vi "Execute_remote_call.vi"(0 "Traverse line":T4 {"Carrier_2 Q (l/min)" format="%#.2f"; "Row Duration (mins)" format="%#.1f"; "Row No" min=0; "Trace Gas Concentration (%)" min=0.0 format="%#_4f"; "Carrier_1 Q (l/min)" format="%#.4f"; "Start X" format="%#.2f"; "Start Y" format="%#.2f"; "Start Z" format="%#.2f"; "End X" format="%#.2f"; "End Y" format="%#.2f"; "End Z" format="%#.2f"; "Tunnel Speed" format="%#.2f"; "Averaging time (mins)" min=0.0 format="%#.2f"}, 2 "Simulate/Run":T3, 3 "VI to run":path) -> (6 "Traverse Out":T4 {"Carrier_2 Q (l/min)" format="%#.2f"; "Row Duration (mins)" format="%#.1f"; "Row No" min=0; "Trace Gas Concentration (%)" min=0.0 format="%#_4f"; "Carrier_1 Q (l/min)" format="%#.4f"; "Start X" format="%#.2f"; "Start Y" format="%#.2f"; "Start Z" format="%#.2f"; "End X" format="%#.2f"; "End Y" format="%#.2f"; "End Z" format="%#.2f"; "Tunnel Speed" format="%#.2f"; "Averaging time (mins)" min=0.0 format="%#.2f"}, 7 "Status":T2, 8 "Error Messages":string)   [LabVIEW 2020]
uses:
  Traverse_cluster.ctl
  Spacing.ctl
  Controls/Multi_run_mode.ctl
  Controls/User_Specific_mode.ctl
  Multi_Run_Status.ctl
  Controls/Multirun_Execute_Row_Connector_Pane.ctl
panel:
  in  "User Specific":T1
  # "X           Y          Z"
  # "Start"
  # "End"
  # "X           Y          Z"
  # "Start"
  # "End"
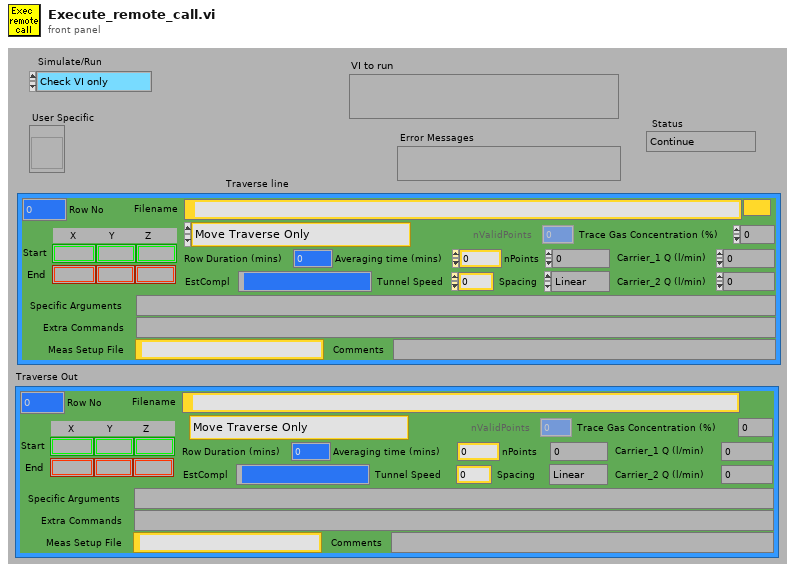
[diagram p1: front panel]
types:
  T1 = typedef "Multirun_Execute_Row_Connector_Pane.ctl" = refnum<vi>
  T2 = typedef "Multi_Run_Status.ctl" = enum16{"Continue", "Continue with Error", "Jump to Next Point", "Jump to Next Row", "Jump To Fall Back", "Terminate Run"}
  T3 = typedef "User_Specific_mode.ctl" = enum16{"Check VI only", "Run VI"}
  T4 = typedef "Traverse_cluster.ctl" = cluster{"Start X":sgl, "Start Y":sgl, "Start Z":sgl, "End X":sgl, "End Y":sgl, "End Z":sgl, "nPoints":i32, "Spacing":T5, "Filename":path, "Tunnel Speed":dbl, "Averaging time (mins)":dbl, "Extra Commands":string, "Carrier_1 Q (l/min)":dbl, "Carrier_2 Q (l/min)":dbl, "Trace Gas Concentration (%)":dbl, "Specific Arguments":string, "Comments":string, "Row No":i32, "Row Type Selector":T6, "EstCompl":string, "Row Duration (mins)":dbl, "nValidPoints":i32, "Meas Setup File":string}
  T5 = typedef "Spacing.ctl" = enum16{"Linear", "Log", "Gauss", "Specified", "N/A"}
  T6 = typedef "Multi_run_mode.ctl" = enum16{"Move Traverse Only", "Set Tunnel Speed Only", "Set Source Only", "Set Measurement Conditions", "Single Measurement", "Vertical Profile", "Lateral Profile", "Longitudinal Profile", "Multi-Axis Profile", "Explore Volume", "Auto Calibrate", "Meas Fast FID Bkgnd", "Check Beam Power", "Scanning Valve Measurement", "Run VI Named:", "Set ADAM Ch", "Wait (minutes)", "Send Message", "Synchronize With:", "Fall Back to this Row", "Turn Off Row Repeating", "Traverse 3D Volume", "Blank Row", "Jump to Fall Back Row"}
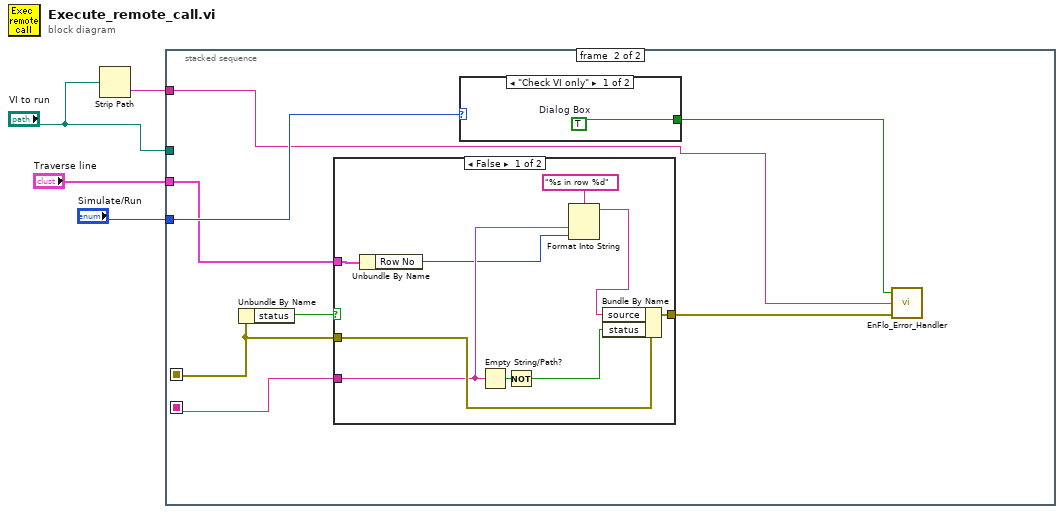
[diagram p0: block diagram]
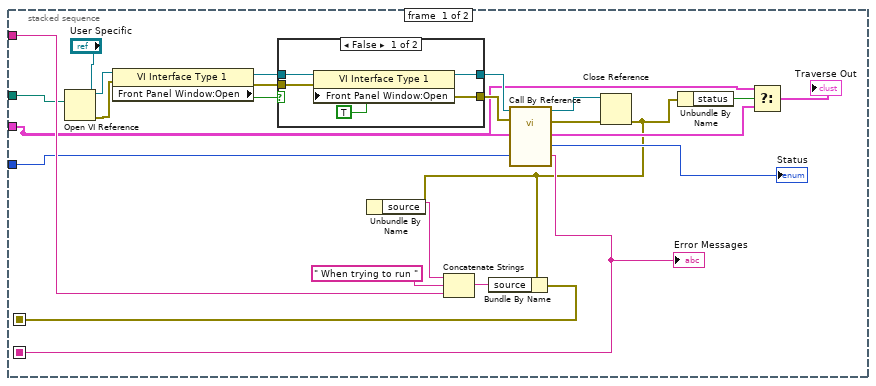
[diagram p2: hidden frame]
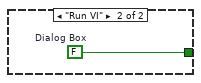
[diagram p4: hidden frame]
diagram:
  n1 = Strip Path(path="VI to run") -> (name=w2:string)  [unwired: 1 out]
  n2 = stacked-sequence {
    seq-local: [w20 _] -> [_ w38]
    seq-local: [w23 _] -> [_ w39]
    tunnel: w2 -> [w24 w36]
    tunnel: "Simulate/Run" -> [w22 w42]
    tunnel: "VI to run" -> [w21 _]
    tunnel: "Traverse line" -> [w6 w37]
    frame #0 {
      n3 = Open VI Reference(type specifier VI Refnum (for type only)="User Specific", vi path=w21) -> (vi reference=w8:T1, error out=w10:errorcluster)  [unwired: 2 in, 2 out]
      n4 = property class="VI Interface Type 1"(reference=w8, error in=w10) -> (reference out=w12:T1, error out=w13:errorcluster, "Front Panel Window:Open"=w11:bool)
      n5 = case shown="False" w11 {
        tunnel: w12 -> [w33 w35]
        tunnel: w13 -> [w32 w34]
        tunnel: [w31 w35] -> w7
        tunnel: [w29 w34] -> w9
        frame False {
          n6 = property class="VI Interface Type 1"(reference=w33, error in=w32, "Front Panel Window:Open"=TRUE) -> (reference out=w31:T1, error out=w29:errorcluster)
        }
        frame True {
        }
      }
      n7 = call-by-ref "?"(reference=w7, error in=w9, "Mode"=w22, "Traverse line In"=w6) -> (reference out=w25:T1, error out=w15:errorcluster, "Error Message"=w20:string, "Status"=→"Status":T2, "Traverse line Out"=w17:T4)  [unwired: 1 in]
      "Error Messages" <- w20
      n8 = Close Reference(reference=w25, error in (no error)=w15) -> (error out=w14:errorcluster)
      n9 = Unbundle By Name(w14) -> ("source"=w28:string)
      n10 = Concatenate Strings(w28, " When trying to run " ("Substring"), w24) -> (w26:string)
      n11 = Bundle By Name(cluster=w14, "source"=w26) -> (w23:errorcluster)
      n12 = Unbundle By Name(w14) -> ("status"=w18:bool)
      n13 = Select(t=w6, s=w18, f=w17) -> (s? t:f=→"Traverse Out":T4)
    }
    frame #1 {
      n14 = Unbundle By Name(w39) -> ("status"=w43:bool)
      n15 = case shown="False" w43 {
        tunnel: [w53 w55] -> w40
        tunnel: w39 -> [w54 w55]
        tunnel: w38 -> [w51 _]
        tunnel: w37 -> [w48 _]
        frame False {
          n16 = Unbundle By Name(w48) -> ("Row No"=w46:i32)
          n17 = Empty String/Path?(string/path=w51) -> (empty?=w52:bool)
          n18 = Not(x=w52) -> (.not. x?=w47:bool)
          n19 = Format Into String(format string="%s in row %d" ("Format String"), w51, w46) -> (resulting string=w49:string)  [unwired: 2 in, 1 out]
          n20 = Bundle By Name(cluster=w54, "source"=w49, "status"=w47) -> (w53:errorcluster)
        }
        frame True {
        }
      }
      n21 = case shown="\"Check VI only\"" w42 {
        tunnel: [w44 w45] -> w41
        frame "Check VI only" {
          w44 = TRUE  # Dialog Box
        }
        frame "Run VI" {
          w45 = FALSE  # Dialog Box
        }
      }
      n22 = call "EnFlo_Error_Handler.vi"("error in (no error)"=w40, "Error Type"=w36, "Dialog Box (F)"=w41) -> ()  [unwired: 3 out]
    }
  }
